vi "JSON__Pars_Table_and_param (SubVI).vi"(8 "error in (no error)":errorcluster, 11 "Data":string) -> (0 "error out":errorcluster, 2 "result string":string, 3 "result string 2":string)   [LabVIEW 2018]
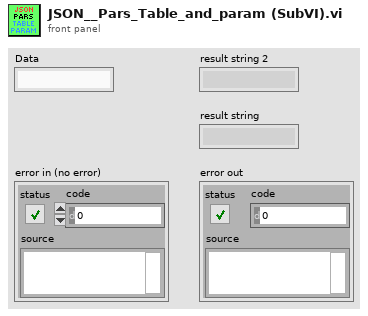
[diagram p1: front panel]
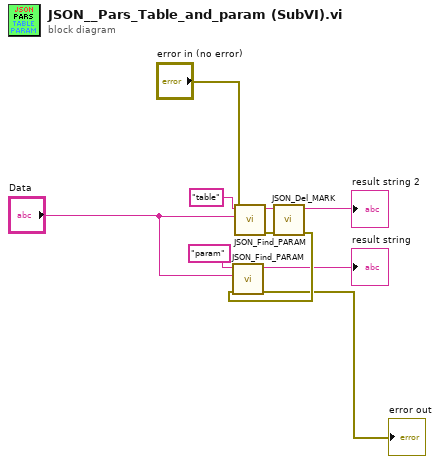
[diagram p0: block diagram]
diagram:
  n1 = call "JSON_Find_PARAM.vi"("error in (no error)"="error in (no error)", "data"="Data", "name"="table") -> ("error out"=w4:errorcluster, "String"=w3:string)  [unwired: 7 in]
  n2 = call "JSON_Del_MARK.vi"("error in (no error)"=w4, "String"=w3) -> ("error out"=w9:errorcluster, "result string"=→"result string 2":string)  [unwired: 8 in]
  n3 = call "JSON_Find_PARAM.vi"("error in (no error)"=w9, "data"="Data", "name"="param") -> ("error out"=→"error out":errorcluster, "String"=→"result string":string)  [unwired: 7 in]
